vi "Stop Core.vi"(10 "final error code":i32, 11 "CS++RTWatchdogActor in":refnum<class "CS++RTWatchdogActor.lvclass">) -> (3 "CS++RTWatchdogActor out":refnum<class "CS++RTWatchdogActor.lvclass">)   [LabVIEW 2016, in "CS++RTWatchdog.lvlib" / "CS++RTWatchdogActor.lvclass"]
doc: "(<B>Filename</B>: Actor Framework.lvlib:Actor.lvclass:Stop Core.vi)\n\nDefines what the actor does before it stops. Use the <B>final error code</B> input to determine whether the actor shut down in response to an error.\n\nBy default, this method does nothing. A descendant class may override it to define behavior, such as shutting down any processes the actor initiated in its override of the Actor Core method."
uses:
  CS++RTWatchdogActor.lvclass
  CS++RTWatchdogActor.lvclass/CS++RTWatchdogActor.ctl
  <vilib>/ActorFramework/Actor/Actor.lvclass
  CSPP_Core/Libraries/Utilities/CS++Utilities.lvlib
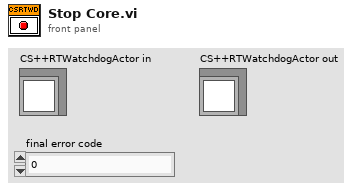
[diagram p1: front panel]
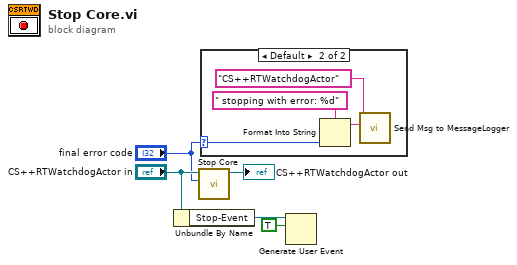
[diagram p0: block diagram]
diagram:
  n1 = Unbundle By Name("CS++RTWatchdogActor in") -> ("Stop-Event"=w3:refnum<user-event>)
  n2 = call-parent "Stop Core.vi"("final error code"="final error code", "Actor in"="CS++RTWatchdogActor in") -> ("Actor out"=→"CS++RTWatchdogActor out":refnum<class "CS++RTWatchdogActor.lvclass">)  [unwired: 9 in]
  n3 = case shown="Default" "final error code" {
    selector: "final error code" -> [_ w8]
    frame 0 {
    }
    frame Default {
      n4 = Format Into String(format string=" stopping with error: %d", w8) -> (resulting string=w7:string)  [unwired: 2 in, 1 out]
      n5 = call "Send Msg to MessageLogger.vi"("Message Content"=w7, "Message Tag"="CS++RTWatchdogActor" ("String to write")) -> ()  [unwired: 9 in, 1 out]
    }
  }
  n6 = Generate User Event(user event=w3, event data cluster=TRUE ("event data")) -> ()  [unwired: 2 in, 2 out]
